vi "Get grpc_reflection_v1alpha_ServerReflectionResponse.vi"(8 "error in (no error)":errorcluster, 11 "gRPCid":T1) -> (0 "error out":errorcluster, 2 "package_templatemessage":T2, 3 "gRPCid out":T1)   [LabVIEW 2025, in "reflection_server.lvlib"]
uses:
  reflection_server.lvlib
  grpc_reflection_v1alpha_ServerReflectionResponse.ctl
  grpc_reflection_v1alpha_ServerReflectionRequest_message_request/grpc_reflection_v1alpha_ServerReflectionRequest_message_request.lvclass
  grpc_reflection_v1alpha_ServerReflectionResponse_message_response/grpc_reflection_v1alpha_ServerReflectionResponse_message_response.lvclass
  grpc_reflection_v1alpha_ServerReflectionRequest.ctl
  <vilib>/gRPC/LabVIEW gRPC Library/Shared/grpcId.ctl
  grpc_reflection_v1alpha_ServerReflectionResponse_Flat.ctl
  grpc_reflection_v1alpha_ServerReflectionRequest_Flat.ctl
  grpc_reflection_v1alpha_ExtensionRequest_Flat.ctl
  grpc_reflection_v1alpha_FileDescriptorResponse_Flat.ctl
  grpc_reflection_v1alpha_ExtensionNumberResponse_Flat.ctl
  grpc_reflection_v1alpha_ListServiceResponse_Flat.ctl
  grpc_reflection_v1alpha_ServiceResponse_Flat.ctl
  grpc_reflection_v1alpha_ErrorResponse_Flat.ctl
  grpc_reflection_v1alpha_ServerReflectionRequest_message_request/grpc_reflection_v1alpha_ServerReflectionRequest_message_request.lvclass/grpc_reflection_v1alpha_ServerReflectionRequest_message_request.ctl
  grpc_reflection_v1alpha_ServerReflectionResponse_message_response/grpc_reflection_v1alpha_ServerReflectionResponse_message_response.lvclass/grpc_reflection_v1alpha_ServerReflectionResponse_message_response.ctl
  2ed25e12-861d-4677-8ead-ace2906b2041.vi
  <vilib>/gRPC/LabVIEW gRPC Library/Shared/TranslateGrpcError.vi
  FlatToRichgrpc_reflection_v1alpha_ServerReflectionRequest.vi
  grpc_reflection_v1alpha_ServerReflectionResponse_message_response/Setfile_descriptor_response.vi
  FlatToRichgrpc_reflection_v1alpha_FileDescriptorResponse.vi
  grpc_reflection_v1alpha_ServerReflectionResponse_message_response/Setall_extension_numbers_response.vi
  FlatToRichgrpc_reflection_v1alpha_ExtensionNumberResponse.vi
  grpc_reflection_v1alpha_ServerReflectionResponse_message_response/Setlist_services_response.vi
  FlatToRichgrpc_reflection_v1alpha_ListServiceResponse.vi
  grpc_reflection_v1alpha_ServerReflectionResponse_message_response/Seterror_response.vi
  FlatToRichgrpc_reflection_v1alpha_ErrorResponse.vi
  grpc_reflection_v1alpha_ServerReflectionRequest_message_request/Setfile_by_filename.vi
  grpc_reflection_v1alpha_ServerReflectionRequest_message_request/Setfile_containing_symbol.vi
  grpc_reflection_v1alpha_ServerReflectionRequest_message_request/Setfile_containing_extension.vi
  FlatToRichgrpc_reflection_v1alpha_ExtensionRequest.vi
  grpc_reflection_v1alpha_ServerReflectionRequest_message_request/Setall_extension_numbers_of_type.vi
  grpc_reflection_v1alpha_ServerReflectionRequest_message_request/Setlist_services.vi
  FlatToRichgrpc_reflection_v1alpha_ServiceResponse.vi
  <vilib>/gRPC/LabVIEW gRPC Library/Server API/Server/Get Server DLL Path.vi
  <vilib>/Utility/error.llb/Error Cluster From Error Code.vi
  grpc_reflection_v1alpha_ServerReflectionResponse_message_response/GetActiveFieldName.vi
  grpc_reflection_v1alpha_ServerReflectionRequest_message_request/GetActiveFieldName.vi
  <vilib>/gRPC/LabVIEW gRPC Library/grpc-lvsupport-release.lvlib
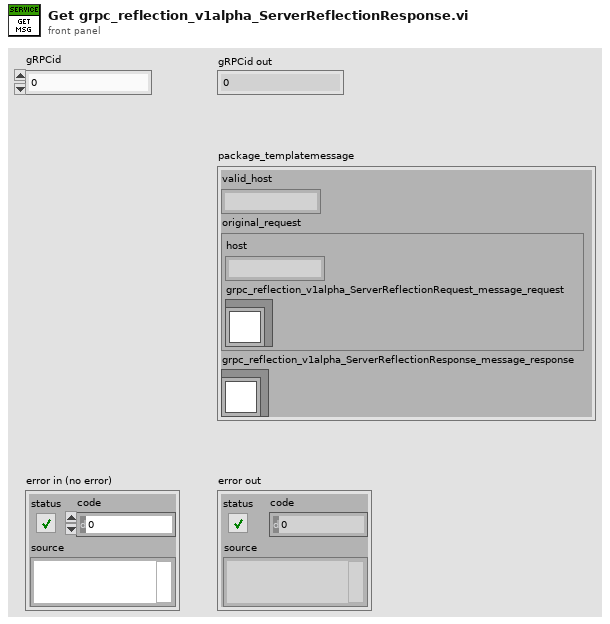
[diagram p1: front panel]
types:
  T1 = typedef "grpc-lvsupport-release.lvlib/grpcId.ctl" = u64
  T2 = typedef "reflection_server.lvlib/grpc_reflection_v1alpha_ServerReflectionResponse.ctl" = cluster{"valid_host":string, "original_request":T3, "grpc_reflection_v1alpha_ServerReflectionResponse_message_response":refnum<class "grpc_reflection_v1alpha_ServerReflectionResponse_message_response.lvclass">}
  T3 = typedef "reflection_server.lvlib/grpc_reflection_v1alpha_ServerReflectionRequest.ctl" = cluster{"host":string, "grpc_reflection_v1alpha_ServerReflectionRequest_message_request":refnum<class "grpc_reflection_v1alpha_ServerReflectionRequest_message_request.lvclass">}
  T4 = typedef "reflection_server.lvlib/grpc_reflection_v1alpha_ServerReflectionResponse_Flat.ctl" = cluster{"valid_host":string, "original_request":T5, "grpc_reflection_v1alpha_ServerReflectionResponse_message_response_selected_index":i32, "file_descriptor_response":T7, "all_extension_numbers_response":T8, "list_services_response":T9, "error_response":T11}
  T5 = typedef "reflection_server.lvlib/grpc_reflection_v1alpha_ServerReflectionRequest_Flat.ctl" = cluster{"host":string, "grpc_reflection_v1alpha_ServerReflectionRequest_message_request_selected_index":i32, "file_by_filename":string, "file_containing_symbol":string, "file_containing_extension":T6, "all_extension_numbers_of_type":string, "list_services":string}
  T6 = typedef "reflection_server.lvlib/grpc_reflection_v1alpha_ExtensionRequest_Flat.ctl" = cluster{"containing_type":string, "extension_number":i32}
  T7 = typedef "reflection_server.lvlib/grpc_reflection_v1alpha_FileDescriptorResponse_Flat.ctl" = cluster{"file_descriptor_proto":cluster{"Array":u8[]}[]}
  T8 = typedef "reflection_server.lvlib/grpc_reflection_v1alpha_ExtensionNumberResponse_Flat.ctl" = cluster{"base_type_name":string, "extension_number":i32[]}
  T9 = typedef "reflection_server.lvlib/grpc_reflection_v1alpha_ListServiceResponse_Flat.ctl" = cluster{"service":T10[]}
  T10 = typedef "reflection_server.lvlib/grpc_reflection_v1alpha_ServiceResponse_Flat.ctl" = cluster{"name":string}
  T11 = typedef "reflection_server.lvlib/grpc_reflection_v1alpha_ErrorResponse_Flat.ctl" = cluster{"error_code":i32, "error_message":string}
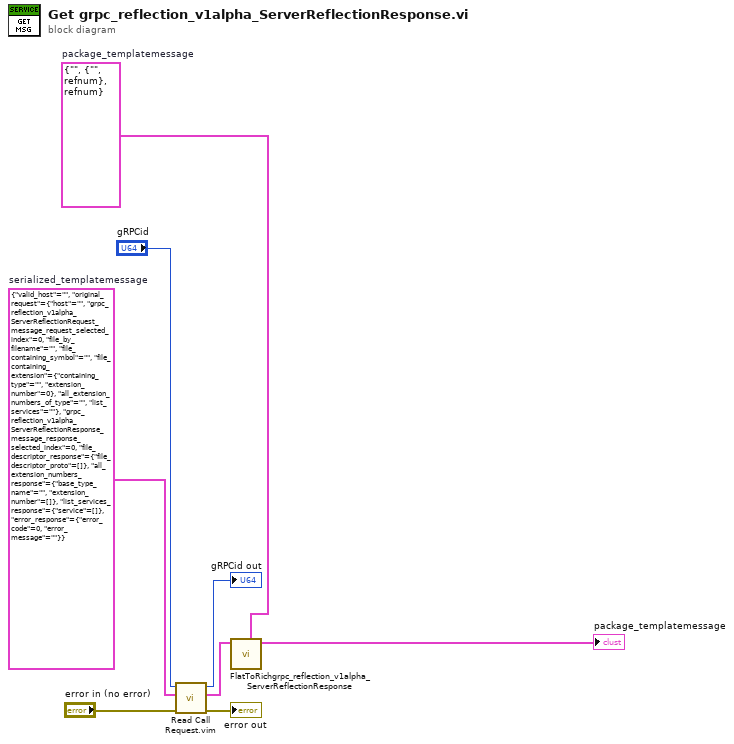
[diagram p0: block diagram]
diagram:
  w6 = T4 {"valid_host"="", "original_request"={"host"="", "grpc_reflection_v1alpha_ServerReflectionRequest_message_request_selected_index"=0, "file_by_filename"="", "file_containing_symbol"="", "file_containing_extension"={"containing_type"="", "extension_number"=0}, "all_extension_numbers_of_type"="", "list_services"=""}, "grpc_reflection_v1alpha_ServerReflectionResponse_message_response_selected_index"=0, "file_descriptor_response"={"file_descriptor_proto"=[]}, "all_extension_numbers_response"={"base_type_name"="", "extension_number"=[]}, "list_services_response"={"service"=[]}, "error_response"={"error_code"=0, "error_message"=""}}  # serialized_templatemessage
  w5 = T2 {"valid_host"="", "original_request"={"host"="", "grpc_reflection_v1alpha_ServerReflectionRequest_message_request"=refnum}, "grpc_reflection_v1alpha_ServerReflectionResponse_message_response"=refnum}  # package_templatemessage
  n1 = call "Read Call Request.vim"("error in"="error in (no error)", "Request Type"=w6, "gRPCid in"="gRPCid") -> ("error out"=→"error out":errorcluster, "Request Data"=w4:T4, "gRPCid out"=→"gRPCid out":T1)  [unwired: 6 in]
  n2 = call "FlatToRichgrpc_reflection_v1alpha_ServerReflectionResponse.vi"("OutputClusterType"=w5, "InputCluster"=w4) -> ("OutputCluster"=→"package_templatemessage":T2)  [unwired: 9 in]
